vi "send_torque_vehicle_command.vi"(4 "error in":errorcluster, 7 "Torque":T1) -> (0 "error out":errorcluster)   [LabVIEW 2019, in "Lib_Simx.lvlib"]
doc: "Sends a command to the Simx Simulator to control the movement of ego vehicle.\n Parameters:\n -- forward_amount: a value between -1.0 and 1.0 that determines the amount of throttle to apply\n -- right_amount: a value between -1.0 and 1.0 that determines the steering position (-1 is left, +1 is right)"
uses:
  Lib_Simx.lvlib
  controls/TorqueControl.ctl
  tools/simx_common.vi
panel:
  out "success":bool
  out "TCP Network Connection out":refnum<k5>
  out "Vehicle command response":string
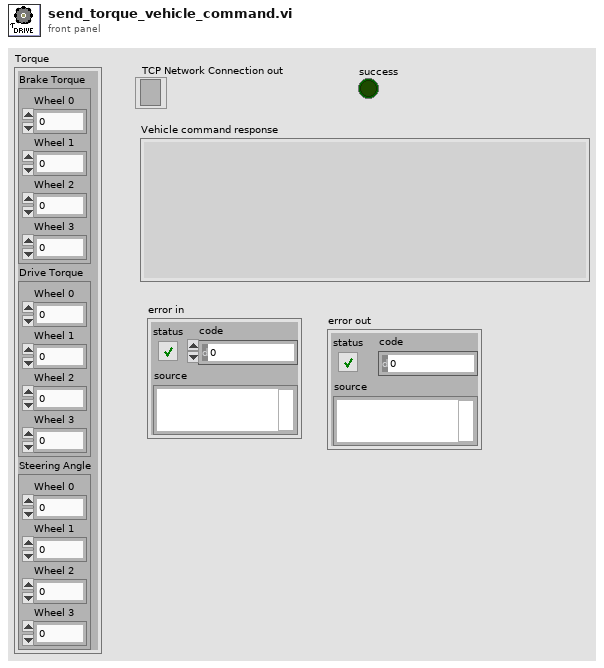
[diagram p1: front panel]
types:
  T1 = cluster{"Brake Torque":cluster{"Wheel 0":sgl, "Wheel 1":sgl, "Wheel 2":sgl, "Wheel 3":sgl}, "Drive Torque":cluster{"Wheel 0":sgl, "Wheel 1":sgl, "Wheel 2":sgl, "Wheel 3":sgl}, "Steering Angle":cluster{"Wheel 0":sgl, "Wheel 1":sgl, "Wheel 2":sgl, "Wheel 3":sgl}}
  T2 = typedef "Lib_Simx.lvlib/simx_connection.ctl" = cluster{"Config":T3, "Connections":T6, "Map":cluster{"lanes":cluster{"x":dbl[], "y":dbl[], "z":dbl[]}, "StartPosition":cluster{"start_points":T7, "StartRotation":dbl[], "StartLocation":dbl[]}, "Draw Map Size":T8, "DrawArea":cluster{"min_Y":dbl, "min_X":dbl, "Scale X":dbl, "Scale Y":dbl}, "Map":picture, "Map Geojson":string}}
  T3 = typedef "Lib_Simx.lvlib/config.ctl" = cluster{"Trajectory":T4, "Weather":T5}
  T4 = typedef "Lib_Simx.lvlib/trajectory.ctl" = cluster{"Number of frames":i32, "Frame number":i32, "Trajectory":string}
  T5 = typedef "Lib_Simx.lvlib/weather.ctl" = cluster{"id":string}
  T6 = typedef "Lib_Simx.lvlib/connections.ctl" = cluster{"Simulator Connection":refnum<k5>, "server_ip":string, "Port":i32, "Sensor connections":refnum<k5>[]}
  T7 = typedef "Lib_Simx.lvlib/start_points.ctl" = cluster{"locations":dbl[][], "rotations":dbl[][], "type":string[]}
  T8 = typedef "LVBoundsTypeDef.ctl" = cluster{"Width":u32, "Height":u32}
  T9 = typedef "Lib_Simx.lvlib/TorqueControl.ctl" = cluster{"brake_torque":sgl[][], "drive_torque":sgl[][], "steer_angle":sgl[][]}
  T10 = cluster{"Wheel 0":sgl, "Wheel 1":sgl, "Wheel 2":sgl, "Wheel 3":sgl}
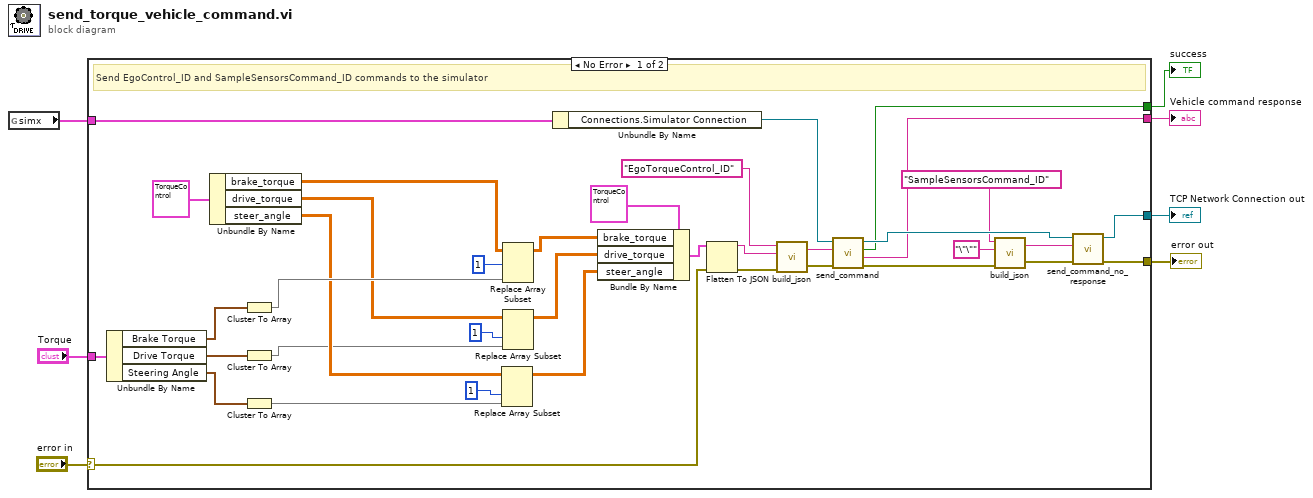
[diagram p0: block diagram]
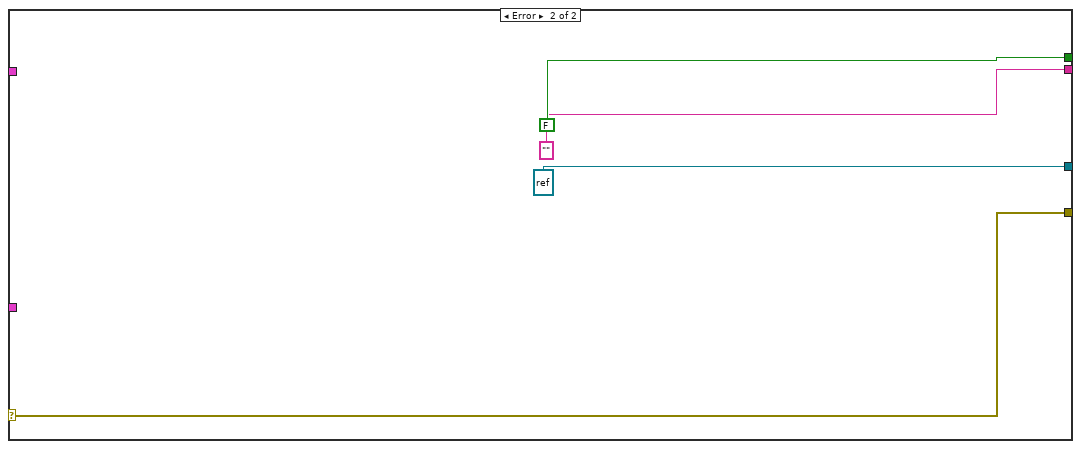
[diagram p2: hidden frame]
diagram:
  n1 = global read "simx_common.vi" "simx"() -> (w2:T2)
  n2 = case shown="No Error" "error in" {
    selector: "error in" -> [w28 w48]
    tunnel: [w38 w48] -> w7
    tunnel: [w34 "" ("response")] -> w6
    tunnel: [w37 refnum<k5> refnum ("TCP Network Connection Out")] -> w5
    tunnel: [w27 FALSE ("success")] -> w4
    tunnel: w2 -> [w44 _]
    tunnel: "Torque" -> [w25 _]
    frame No Error {
      # "Send EgoControl_ID and SampleSensorsCommand_ID commands to the simulator"
      n3 = Unbundle By Name(w25) -> ("Brake Torque"=w24:T10, "Drive Torque"=w20:T10, "Steering Angle"=w19:T10)
      n4 = Unbundle By Name(T9 {"brake_torque"=[[0.0, 0.0], [1.0, 0.0], [2.0, 0.0], [3.0, 0.0]], "drive_torque"=[[0.0, 500000.0], [1.0, 500000.0], [2.0, 0.0], [3.0, 0.0]], "steer_angle"=[[0.0, 0.0], [1.0, 0.0], [2.0, 0.0], [3.0, 0.0]]} ("TorqueControl")) -> ("brake_torque"=w26:sgl[][], "drive_torque"=w18:sgl[][], "steer_angle"=w17:sgl[][])
      n5 = Cluster To Array(cluster=w24) -> (array=w23:sgl[])
      n6 = Cluster To Array(cluster=w20) -> (array=w12:sgl[])
      n7 = Cluster To Array(cluster=w19) -> (array=w13:sgl[])
      n8 = Replace Array Subset(array=w17, new element=w13, index (col)=1 ("disabled index (col)")) -> (w10:sgl[][])  [unwired: 1 in]
      n9 = Replace Array Subset(array=w26, new element=w23, index (col)=1 ("disabled index (col)")) -> (w22:sgl[][])  [unwired: 1 in]
      n10 = Replace Array Subset(array=w18, new element=w12, index (col)=1 ("disabled index (col)")) -> (w11:sgl[][])  [unwired: 1 in]
      n11 = Unbundle By Name(w44) -> ("Connections.Simulator Connection"=w42:refnum<k5>)
      n12 = Bundle By Name(cluster=T9 {"brake_torque"=[[0.0, 0.0], [1.0, 0.0], [2.0, 0.0], [3.0, 0.0]], "drive_torque"=[[0.0, 500000.0], [1.0, 500000.0], [2.0, 0.0], [3.0, 0.0]], "steer_angle"=[[0.0, 0.0], [1.0, 0.0], [2.0, 0.0], [3.0, 0.0]]} ("TorqueControl"), "brake_torque"=w22, "drive_torque"=w11, "steer_angle"=w10) -> (w21:T9)
      n13 = Flatten To JSON(anything=w21, error in (no error)=w28) -> (JSON string=w30:string, 11:w31:errorcluster)  [unwired: 1 in]
      n14 = call "build_json.vi"("error in"=w31, "Message"=w30, "Command_ID"="EgoTorqueControl_ID") -> ("error out"=w43:errorcluster, "JSON Out"=w41:string)  [unwired: 1 in]
      n15 = call "send_command.vi"("error in"=w43, "JSON Command"=w41, "TCP Network Connection in"=w42) -> ("error out"=w40:errorcluster, "Response"=w34:string, "Success"=w27:bool, "TCP Network Connection Out"=w35:refnum<k5>)  [unwired: 1 in]
      n16 = call "build_json.vi"("error in"=w40, "Message"="\"\"" ("message"), "Command_ID"="SampleSensorsCommand_ID" ("type")) -> ("error out"=w39:errorcluster, "JSON Out"=w36:string)  [unwired: 1 in]
      n17 = call "send_command_no_response.vi"("error in"=w39, "JSON Command"=w36, "TCP Network Connection in"=w35) -> ("error out"=w38:errorcluster, "TCP Network Connection Out"=w37:refnum<k5>)  [unwired: 3 in]
    }
    frame Error {
    }
  }
  "Vehicle command response" <- w6
  "TCP Network Connection out" <- w5
  "error out" <- w7
  "success" <- w4
